vi "Build Measurement.vi"() -> ()   [LabVIEW 2021]
uses:
  <vilib>/Utility/miscctls.llb/LVRowAndColumnTypeDef.ctl
  _Measurement Packager Utility/Packager Helpers/Queue Driver/controls/Queue Operations.ctl
  _Measurement Packager Utility/Packager Helpers/controls/Config File Operations.ctl
  _Measurement Packager Utility/Packager Helpers/controls/Data Holder.ctl
  <vilib>/Utility/miscctls.llb/LVPoint32TypeDef.ctl
  _Measurement Packager Utility/Packager Helpers/controls/Build Spec Details.ctl
  <vilib>/AppBuilder/AB_API_Simple/Get Build Specification Version (path).vi
  _Measurement Packager Utility/Packager Helpers/Queue Driver/Queue Driver.lvlib
  _Measurement Packager Utility/Packager Helpers/Packager Helpers.lvlib
  _Measurement Packager Utility/Packager Helpers/Dictionary/Dictionary.lvlib
  <vilib>/AppBuilder/AB_API_Simple/NI_App_Builder_API.lvlib
panel:
  out "error out":errorcluster
  out "Tab Control":T1(tab)
  in  "Open Directory":bool
  in  "Feed Path":path
  out "Warning":bool=TRUE caption="Feed Path cannot be empty/invalid"
  in  "Next to select":bool
  in  "Build Package":bool
  in  "Project":path caption="LabVIEW Project Path"
  in  "Feed":T2(radio)
  in  "Back 1":bool
  in  "Populate Package":bool
  in  "Select All":bool
  out "Measurement List":i32(listbox)=-1 caption="Select the Measurements to build the package"
  out "Selection warning":string="Selected Project doesn't have EXE build spec"
  out "Maintainer Warning":string
  in  "Settings Page":enum32{"Page 1", "Page 2"}(tab)
  in  "Maintainer Email ID":string="sabthagiri@ni.com"
  in  "Architecture":string(combo)="1"
  in  "Maintainer":string="NI"
  in  "Back 2":bool
  in  "Start Build":bool
  in  "Package List":i32[](listbox) caption="Edit the Package Name and Version"
  in  "Settings":bool
  in  "Progres Bar":i32(slide)=9 caption="Creating Distribution..." scale=0.0..100.0
  in  "Start Next":bool
  in  "Log":bool[](array[boolean])=[TRUE, TRUE]
  in  "Build Status":i32(listbox)=-1
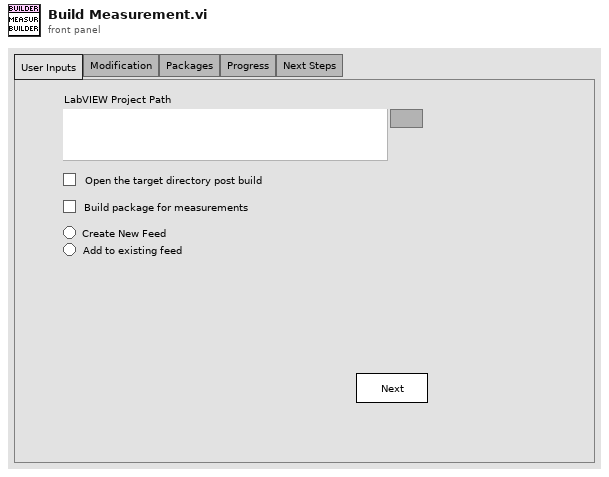
[diagram p1: front panel]
types:
  T1 = enum32{"User Inputs", "Modification", "Packages", "Progress", "Next Steps"}
  T2 = enum32{"No Selection", "CreateFeed", "AddtoFeed"}
  T3 = typedef "Queue Driver.lvlib/Queue Operations.ctl" = enum16{"Create Q", "Enqueue", "Enqueue N", "Dequeue", "Flush", "Release"}
  T4 = typedef "LVRowAndColumnTypeDef.ctl" = cluster{"Row":i32, "Column":i32}
  T5 = enum8{"Enabled", "Disabled", "Disabled and Grayed Out"}
  T6 = typedef "Packager Helpers.lvlib/Config File Operations.ctl" = enum16{"Read", "Write"}
  T7 = typedef "Packager Helpers.lvlib/Data Holder.ctl" = cluster{"Next Clicked?":bool, "MosueDown Coords":T8, "Build Spec":T9[], "No of Meas":i32, "No. of Selected Meas":i32, "Selected Meas":T9[], "Package Details":string[][], "Build Packge?":bool, "Packages Path":path, "Feed":enum32{"No Selection", "CreateFeed", "AddtoFeed"}, "Feed Path":path, "Valid Inputs?":bool, "Feed Old":enum32{"No Selection", "CreateFeed", "AddtoFeed"}, "Status":string[], "Open Directory?":bool}
  T8 = typedef "LVPoint32TypeDef.ctl" = cluster{"Horizontal":i32, "Vertical":i32}
  T9 = typedef "Packager Helpers.lvlib/Build Spec Details.ctl" = cluster{"EXE Name":string, "Target path":path, "Has PPL?":bool, "PPL Name":string}
  T10 = typedef "NI_App_Builder_API.lvlib/Build Specification Version.ctl" = cluster{"Major":u16, "Minor":u16, "Fix":u16, "Build":u16}
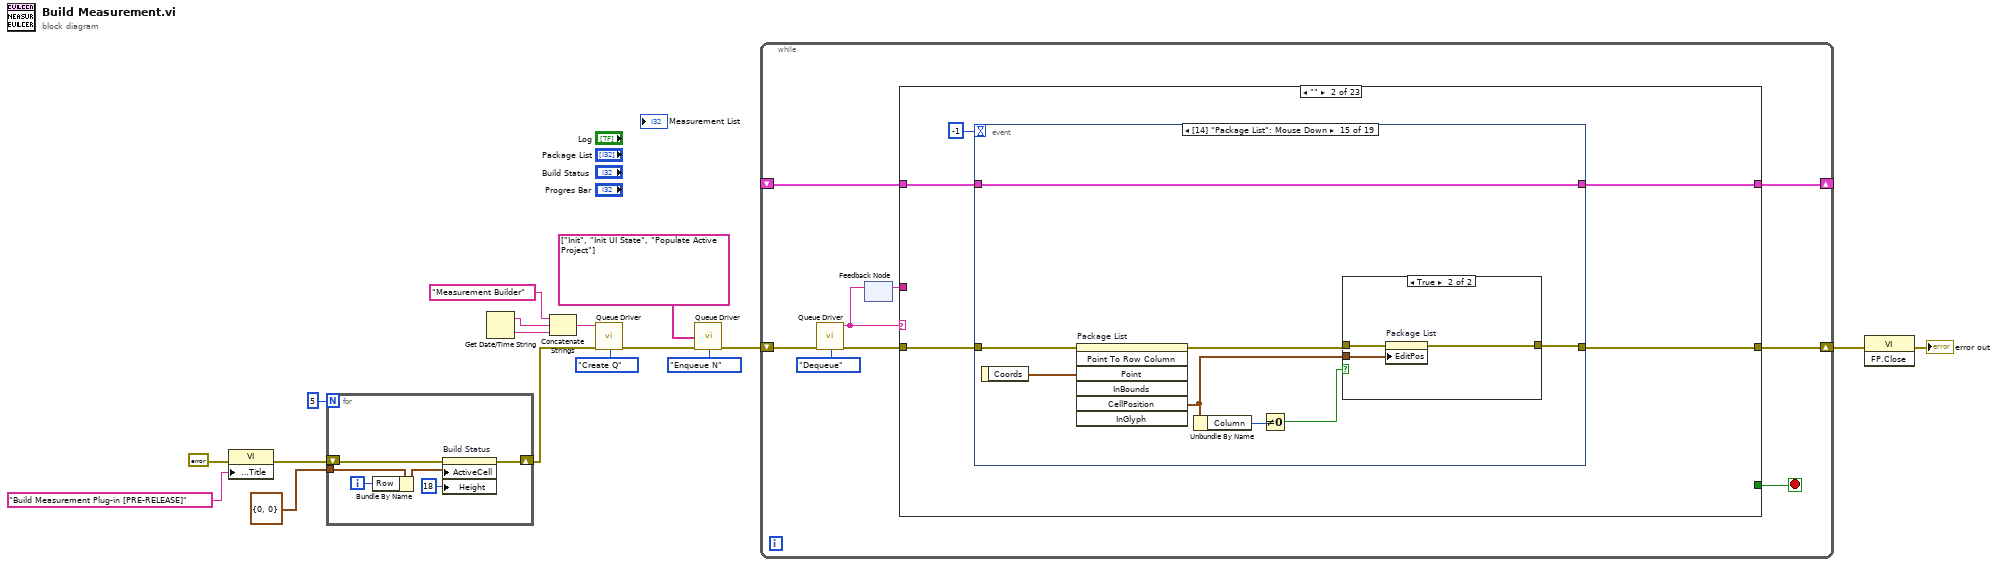
[diagram p0: block diagram]
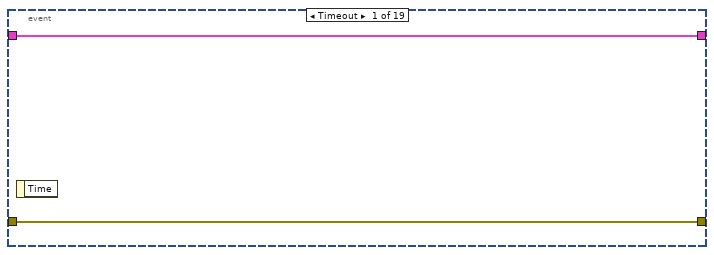
[diagram p3: hidden frame]
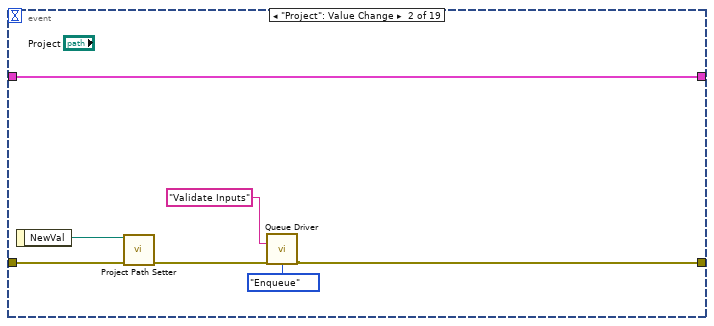
[diagram p4: hidden frame]
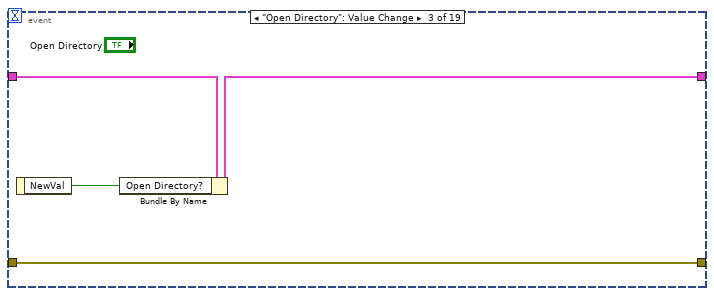
[diagram p5: hidden frame]
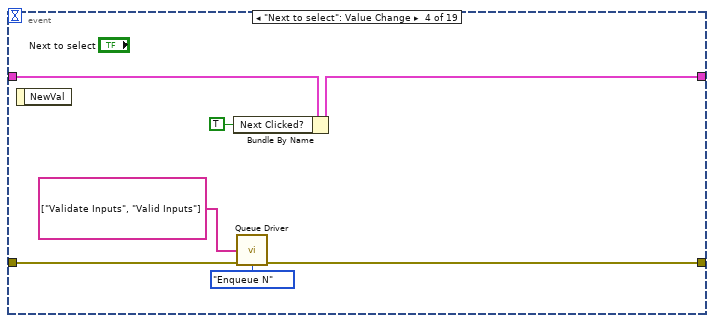
[diagram p6: hidden frame]
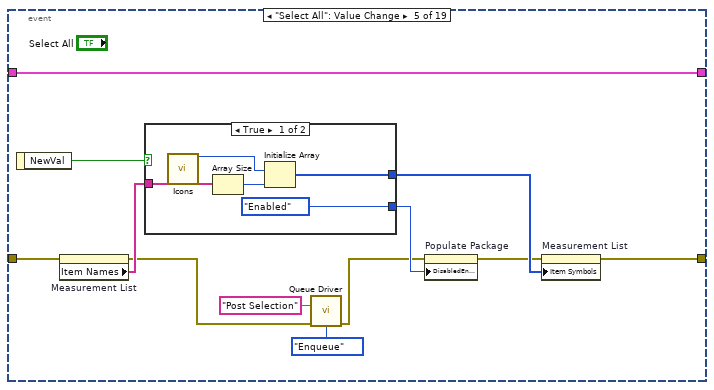
[diagram p7: hidden frame]
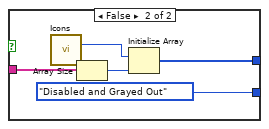
[diagram p8: hidden frame]
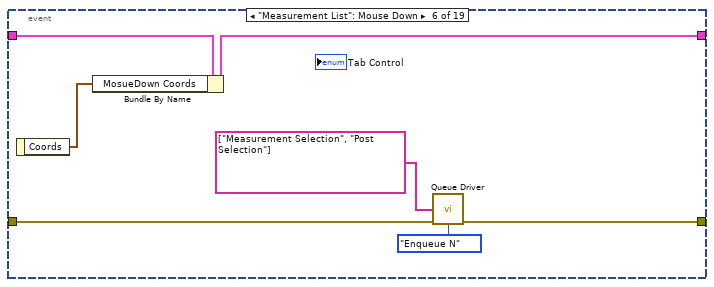
[diagram p9: hidden frame]
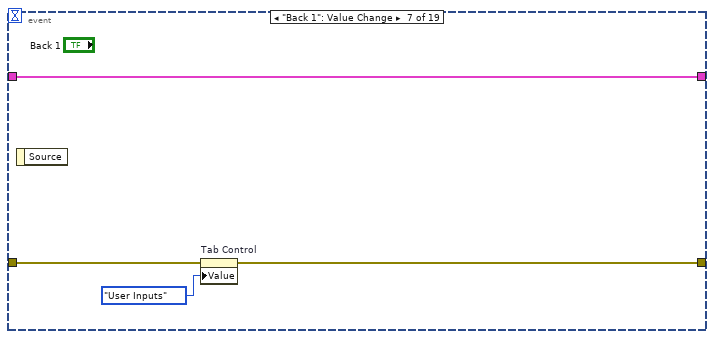
[diagram p10: hidden frame]
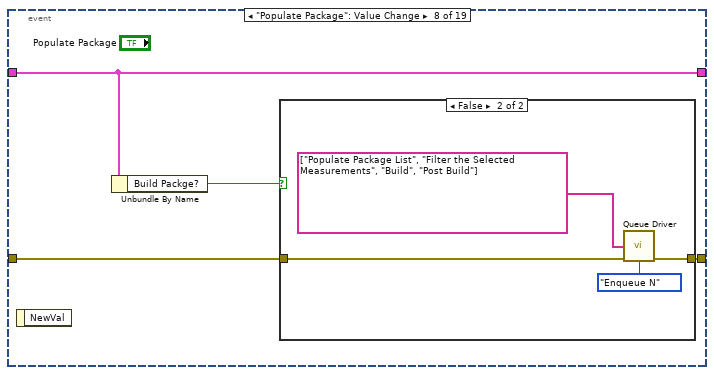
[diagram p11: hidden frame]
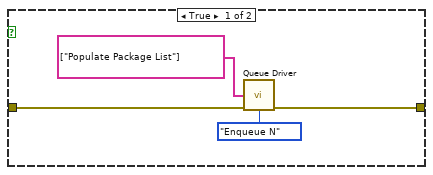
[diagram p12: hidden frame]
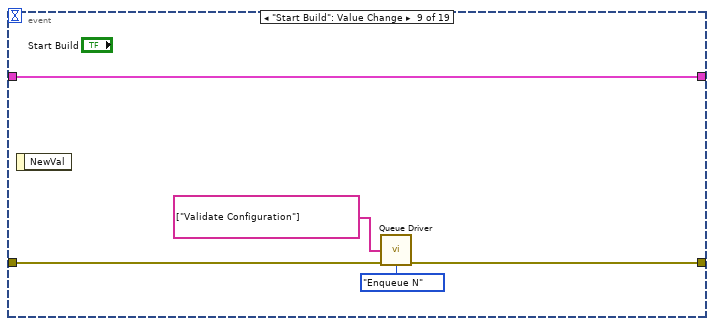
[diagram p13: hidden frame]
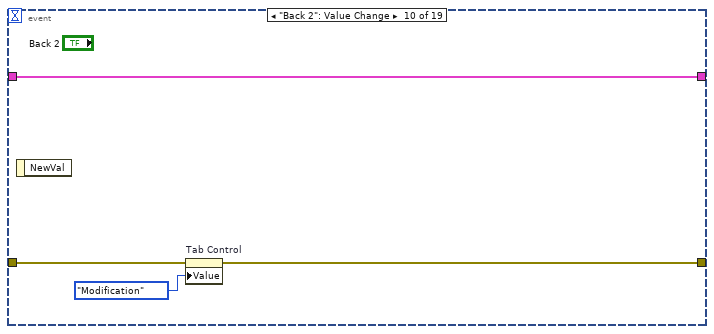
[diagram p14: hidden frame]
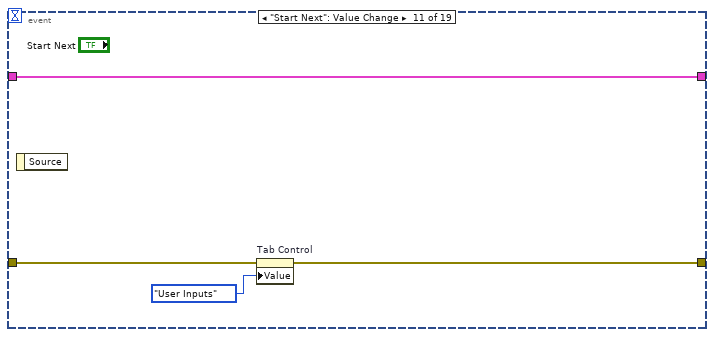
[diagram p15: hidden frame]
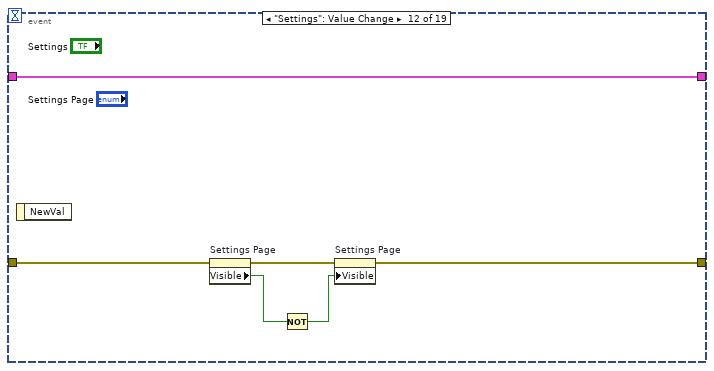
[diagram p16: hidden frame]
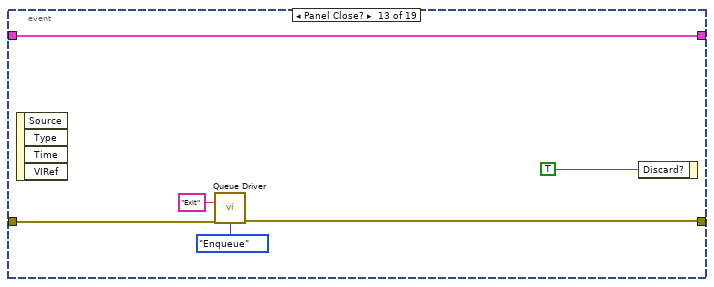
[diagram p17: hidden frame]
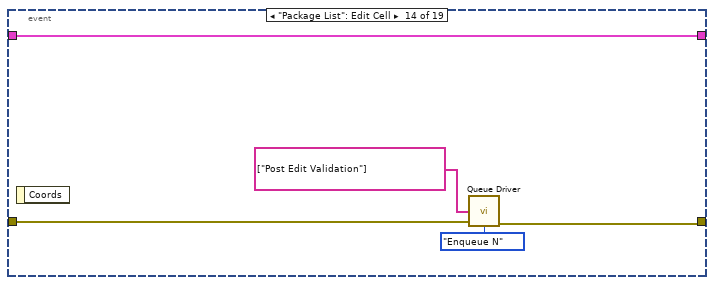
[diagram p18: hidden frame]
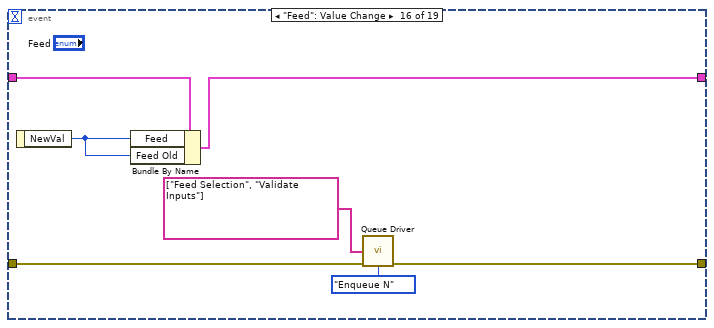
[diagram p20: hidden frame]
diagram:
  n1 = property class="VI"(error in=errorcluster {"status"=FALSE, "code"=0, "source"=""} ("error in (no error)"), "Front Panel.Title"="Build Measurement Plug-in [PRE-RELEASE]" ("Front Panel Window:Title")) -> (error out=w3:errorcluster)  [unwired: 1 in, 1 out]
  n2 = for {
    N: 5 -> [_]
    tunnel: T4 {"Row"=0, "Column"=0} ("Active Cell:Active Cell") -> [w23]
    shift-right: [w19] -> w6
    shift-left: w3 -> [w18]
    i -> [w21]
    n3 = Bundle By Name(cluster=w23, "Row"=w21) -> (w22:T4)
    n4 = property on="Build Status" class="MCListbox (strict)"(error in=w18, "ActiveCell"=w22, "Height"=u32 18 ("Active Cell:Cell Size:Height")) -> (error out=w19:errorcluster)  [unwired: 1 in, 1 out]
  }
  n5 = Get Date/Time String() -> (date string=w9:string, time string=w10:string)  [unwired: 3 in]
  n6 = Concatenate Strings("Measurement Builder" ("string"), w9, w10) -> (w7:string)
  n7 = call "Queue Driver.vi"("Name"=w7, "error in (no error)"=w6, "Q Operations"=Queue_Operations."Create Q") -> ("error out"=w13:errorcluster)  [unwired: 11 in, 1 out]
  n8 = call "Queue Driver.vi"("States[]"=string[] ["Init", "Init UI State", "Populate Active Project"], "error in (no error)"=w13, "Q Operations"=Queue_Operations."Enqueue N") -> ("error out"=w15:errorcluster)  [unwired: 11 in, 1 out]
  n9 = while {
    shift-right: [w29] -> w5
    shift-left: w15 -> [w32]
    shift-right: [w27] -> _
    shift-left: _ -> [w26]
    stop <- w28 stop-if-true
    n10 = call "Queue Driver.vi"("error in (no error)"=w32, "Q Operations"=Queue_Operations."Dequeue") -> ("Dequeued State"=w25:string, "error out"=w30:errorcluster)  [unwired: 12 in]
    n11 = feedback #1() -> (w24:string)  [unwired: 1 in]
    n12 = feedback-in #1(w25) -> ()
    n13 = case shown="\"\"" w25 {
      tunnel: w30 -> [w34 w38 w179 w194 w213 w225 w242 w291 w306 w328 w342 w367 w393 w399 w408 w433 w462 w472 w487 w506 w509 w526 w532]
      tunnel: [w34 w39 w176 w188 w206 w224 w239 w290 w309 w326 w338 w359 w388 w400 w405 w427 w461 w468 w478 w507 w515 w525 w531] -> w29
      tunnel: [_ _ _ _ _ _ _ _ _ _ _ _ _ _ _ _ _ _ _ _ _ _ TRUE] -> w28
      tunnel: [w33 w36 w178 w190 w209 w226 w238 w289 w311 w329 w345 w368 w391 w401 w412 w424 w463 w464 w488 w505 w514 w527 w528] -> w27
      tunnel: w26 -> [w33 w35 _ w190 w210 w226 w237 w289 w312 w329 w345 w368 w394 w401 w412 w421 w463 w466 w488 w499 w514 w527 w528]
      tunnel: w24 -> [_ _ _ _ _ _ _ _ _ _ _ _ _ _ _ _ _ _ _ _ _ _ _]
      frame Default {
      }
      frame "" {
        n14 = event shown="[14] \"Package List\": Mouse Down" {
          selector: _ -> [_ _ _ _ _ _ _ _ _ _ _ _ _ _ _ _ _ _ _]
          dyn-events: _ -> [_ _ _ _ _ _ _ _ _ _ _ _ _ _ _ _ _ _ _]
          timeout: -1 -> [_ _ _ _ _ _ _ _ _ _ _ _ _ _ _ _ _ _ _]
          tunnel: [w41 w44 w52 w58 w64 w85 w91 w95 w107 w112 w116 w120 w127 w132 w135 w150 w156 w165 w168] -> w39
          tunnel: w38 -> [w41 w48 w52 w59 w69 w87 w92 w96 w108 w113 w117 w121 w128 w130 w140 w149 w155 w164 w169]
          tunnel: [w40 w42 w50 w55 w71 w84 w90 w94 w109 w111 w115 w118 w124 w134 w142 w152 w159 w167 w173] -> w36
          tunnel: w35 -> [w40 w42 w51 w56 w71 w88 w90 w94 w109 w111 w115 w118 w124 w134 w142 w153 w160 w167 w174]
          event Timeout {
            n15 = event-data() -> ()  [unwired: 1 in, 1 out]
          }
          event "Project": Value Change {
            n16 = event-data() -> ("NewVal"=w47:path)  [unwired: 1 in]
            n17 = call "Project Path Setter.vi"("ProjectPath In"=w47, "error in (no error)"=w48) -> ("error out"=w43:errorcluster)  [unwired: 13 in]
            n18 = call "Queue Driver.vi"("State"="Validate Inputs", "error in (no error)"=w43, "Q Operations"=Queue_Operations."Enqueue") -> ("error out"=w44:errorcluster)  [unwired: 11 in, 1 out]
          }
          event "Open Directory": Value Change {
            n19 = event-data() -> ("NewVal"=w49:bool)  [unwired: 1 in]
            n20 = Bundle By Name(cluster=w51, "Open Directory?"=w49) -> (w50:T7)
          }
          event "Next to select": Value Change {
            n21 = event-data() -> ()  [unwired: 1 in, 1 out]
            n22 = Bundle By Name(cluster=w56, "Next Clicked?"=TRUE) -> (w55:T7)
            n23 = call "Queue Driver.vi"("States[]"=string[] ["Validate Inputs", "Valid Inputs"], "error in (no error)"=w59, "Q Operations"=Queue_Operations."Enqueue N") -> ("error out"=w58:errorcluster)  [unwired: 11 in, 1 out]
          }
          event "Select All": Value Change {
            n24 = event-data() -> ("NewVal"=w70:bool)  [unwired: 1 in]
            n25 = property on="Measurement List" class="LstBox (strict)"(error in=w69) -> (error out=w61:errorcluster, "Item Names"=w68:string[])  [unwired: 1 in, 1 out]
            n26 = case shown="True" w70 {
              tunnel: w68 -> [w75 w80]
              tunnel: [w74 w79] -> w67
              tunnel: [T5."Enabled" ("Disabled") T5."Disabled and Grayed Out" ("Disabled")] -> w66
              frame True {
                n27 = call "Icons.vi"() -> ("Selected"=w72:i32)  [unwired: 14 in, 1 out]
                n28 = Array Size(array=w75) -> (size(s)=w76:i32)
                n29 = Initialize Array(w72, w76) -> (w74:i32[])
              }
              frame False {
                n30 = call "Icons.vi"() -> ("Non Selected"=w77:i32)  [unwired: 14 in, 1 out]
                n31 = Array Size(array=w80) -> (size(s)=w81:i32)
                n32 = Initialize Array(w77, w81) -> (w79:i32[])
              }
            }
            n33 = call "Queue Driver.vi"("State"="Post Selection", "error in (no error)"=w61, "Q Operations"=Queue_Operations."Enqueue") -> ("error out"=w60:errorcluster)  [unwired: 11 in, 1 out]
            n34 = property on="Populate Package" class="Bool"(error in=w60, "DisabledEnum"=w66) -> (error out=w65:errorcluster)  [unwired: 1 in, 1 out]
            n35 = property on="Measurement List" class="LstBox (strict)"(error in=w65, "Item Symbols"=w67) -> (error out=w64:errorcluster)  [unwired: 1 in, 1 out]
          }
          event "Measurement List": Mouse Down {
            n36 = event-data() -> ("Coords"=w82:T8)  [unwired: 1 in]
            n37 = Bundle By Name(cluster=w88, "MosueDown Coords"=w82) -> (w84:T7)
            n38 = call "Queue Driver.vi"("States[]"=string[] ["Measurement Selection", "Post Selection"], "error in (no error)"=w87, "Q Operations"=Queue_Operations."Enqueue N") -> ("error out"=w85:errorcluster)  [unwired: 11 in, 1 out]
          }
          event "Back 1": Value Change {
            n39 = event-data() -> ()  [unwired: 1 in, 1 out]
            n40 = property on="Tab Control" class="TabCtl (strict)"(error in=w92, "Value"=T1."User Inputs" ("Tab Control")) -> (error out=w91:errorcluster)  [unwired: 1 in, 1 out]
          }
          event "Populate Package": Value Change {
            n41 = event-data() -> ()  [unwired: 1 in, 1 out]
            n42 = Unbundle By Name(w94) -> ("Build Packge?"=w93:bool)
            n43 = case shown="False" w93 {
              tunnel: w96 -> [w100 w104]
              tunnel: [w99 w103] -> w95
              frame True {
                n44 = call "Queue Driver.vi"("States[]"=string[] ["Populate Package List"], "error in (no error)"=w100, "Q Operations"=Queue_Operations."Enqueue N") -> ("error out"=w99:errorcluster)  [unwired: 11 in, 1 out]
              }
              frame False {
                n45 = call "Queue Driver.vi"("States[]"=string[] ["Populate Package List", "Filter the Selected Measurements", "Build", "Post Build"], "error in (no error)"=w104, "Q Operations"=Queue_Operations."Enqueue N") -> ("error out"=w103:errorcluster)  [unwired: 11 in, 1 out]
              }
            }
          }
          event "Start Build": Value Change {
            n46 = event-data() -> ()  [unwired: 1 in, 1 out]
            n47 = call "Queue Driver.vi"("States[]"=string[] ["Validate Configuration"], "error in (no error)"=w108, "Q Operations"=Queue_Operations."Enqueue N") -> ("error out"=w107:errorcluster)  [unwired: 11 in, 1 out]
          }
          event "Back 2": Value Change {
            n48 = event-data() -> ()  [unwired: 1 in, 1 out]
            n49 = property on="Tab Control" class="TabCtl (strict)"(error in=w113, "Value"=T1."Modification" ("Tab Control")) -> (error out=w112:errorcluster)  [unwired: 1 in, 1 out]
          }
          event "Start Next": Value Change {
            n50 = event-data() -> ()  [unwired: 1 in, 1 out]
            n51 = property on="Tab Control" class="TabCtl (strict)"(error in=w117, "Value"=T1."User Inputs" ("Tab Control")) -> (error out=w116:errorcluster)  [unwired: 1 in, 1 out]
          }
          event "Settings": Value Change {
            n52 = event-data() -> ()  [unwired: 1 in, 1 out]
            n53 = property on="Settings Page" class="TabCtl (strict)"(error in=w121) -> (error out=w119:errorcluster, "Visible"=w123:bool)  [unwired: 1 in, 1 out]
            n54 = Not(x=w123) -> (.not. x?=w122:bool)
            n55 = property on="Settings Page" class="TabCtl (strict)"(error in=w119, "Visible"=w122) -> (error out=w120:errorcluster)  [unwired: 1 in, 1 out]
          }
          event Panel Close? {
            n56 = event-data() -> ()  [unwired: 1 in, 4 out]
            n57 = call "Queue Driver.vi"("State"="Exit", "error in (no error)"=w128, "Q Operations"=Queue_Operations."Enqueue") -> ("error out"=w127:errorcluster)  [unwired: 11 in, 1 out]
            n58 = event-data("Discard?"=TRUE) -> ()  [unwired: 1 in, 1 out]
          }
          event "Package List": Edit Cell {
            n59 = event-data() -> ()  [unwired: 1 in, 1 out]
            n60 = call "Queue Driver.vi"("States[]"=string[] ["Post Edit Validation"], "error in (no error)"=w130, "Q Operations"=Queue_Operations."Enqueue N") -> ("error out"=w132:errorcluster)  [unwired: 11 in, 1 out]
          }
          event "Package List": Mouse Down {
            n61 = event-data() -> ("Coords"=w141:T8)  [unwired: 1 in]
            n62 = invoke on="Package List" class="MCListbox (strict)" method="Point To Row Column"(error in=w140, "Point"=w141) -> (error out=w139:errorcluster, "CellPosition"=w136:T4)  [unwired: 5 in, 5 out]
            n63 = Unbundle By Name(w136) -> ("Column"=w138:i32)
            n64 = Not Equal To 0?(x=w138) -> (x != 0?=w137:bool)
            n65 = case shown="True" w137 {
              tunnel: w139 -> [w143 w146]
              tunnel: [w143 w145] -> w135
              tunnel: w136 -> [_ w144]
              frame False {
              }
              frame True {
                n66 = property on="Package List" class="MCListbox (strict)"(error in=w146, "EditPos"=w144) -> (error out=w145:errorcluster)  [unwired: 1 in, 1 out]
              }
            }
          }
          event "Feed": Value Change {
            n67 = event-data() -> ("NewVal"=w147:T2)  [unwired: 1 in]
            n68 = Bundle By Name(cluster=w153, "Feed"=w147, "Feed Old"=w147) -> (w152:T7)
            n69 = call "Queue Driver.vi"("States[]"=string[] ["Feed Selection", "Validate Inputs"], "error in (no error)"=w149, "Q Operations"=Queue_Operations."Enqueue N") -> ("error out"=w150:errorcluster)  [unwired: 11 in, 1 out]
          }
          event "Build Package": Value Change {
            n70 = event-data() -> ("NewVal"=w158:bool)  [unwired: 1 in]
            n71 = Bundle By Name(cluster=w160, "Build Packge?"=w158) -> (w159:T7)
            n72 = call "Queue Driver.vi"("States[]"=string[] ["Build Package Value Change", "Validate Inputs"], "error in (no error)"=w155, "Q Operations"=Queue_Operations."Enqueue N") -> ("error out"=w156:errorcluster)  [unwired: 11 in, 1 out]
          }
          event "Architecture", "Maintainer", "Maintainer Email ID": Value Change {
            n73 = event-data() -> ()  [unwired: 1 in, 1 out]
            n74 = call "Read or Write Configurations.vi"("Architecture"="Architecture", "Maintainer"="Maintainer", "Email"="Maintainer Email ID", "error in (no error)"=w164, "Operation"=Config_File_Operations."Write") -> ("error out"=w165:errorcluster)  [unwired: 7 in, 3 out]
          }
          event "Feed Path": Value Change {
            n75 = event-data() -> ("NewVal"=w172:path)  [unwired: 1 in]
            n76 = Bundle By Name(cluster=w174, "Feed Path"=w172) -> (w173:T7)
            n77 = call "Queue Driver.vi"("States[]"=string[] ["Validate Inputs"], "error in (no error)"=w169, "Q Operations"=Queue_Operations."Enqueue N") -> ("error out"=w168:errorcluster)  [unwired: 11 in, 1 out]
          }
        }
      }
      frame "Init" {
        w177 = TRUE ("Open Directory?")
        n78 = invoke class="VI" method="Default Vals.Reinit All"(error in=w179) -> (error out=w175:errorcluster)  [unwired: 2 in, 2 out]
        n79 = property on="Open Directory" class="Bool (strict)"(error in=w175, "Value"=w177) -> (error out=w176:errorcluster)  [unwired: 1 in, 1 out]
        n80 = Bundle By Name(cluster=T7 {"Next Clicked?"=TRUE, "MosueDown Coords"={"Horizontal"=0, "Vertical"=0}, "Build Spec"=[], "No of Meas"=0, "No. of Selected Meas"=0, "Selected Meas"=[], "Package Details"=[], "Build Packge?"=FALSE, "Packages Path"=path "", "Feed"=enum."No Selection", "Feed Path"=path "", "Valid Inputs?"=FALSE, "Feed Old"=enum."No Selection", "Status"=[], "Open Directory?"=FALSE}, "Open Directory?"=w177) -> (w178:T7)
      }
      frame "Init UI State" {
        w187 = u32 16448250 ("Selection Color")
        w184 = FALSE ("Visible")
        n81 = property on="Tab Control" class="TabCtl (strict)"(error in=w194, "Value"=T1."User Inputs" ("Tab Control")) -> (error out=w197:errorcluster)  [unwired: 1 in, 1 out]
        n82 = property on="Settings Page" class="TabCtl (strict)"(error in=w197, "Visible"=w184) -> (error out=w196:errorcluster)  [unwired: 1 in, 1 out]
        n83 = property on="Warning" class="Bool"(error in=w196, "Visible"=w184) -> (error out=w181:errorcluster)  [unwired: 1 in, 1 out]
        n84 = property on="Selection warning" class="Str"(error in=w181, "Visible"=w184) -> (error out=w186:errorcluster)  [unwired: 1 in, 1 out]
        n85 = property on="Feed Path" class="Path"(error in=w186, "Visible"=w184) -> (error out=w185:errorcluster)  [unwired: 1 in, 1 out]
        n86 = property on="Settings" class="Bool"(error in=w185, "Visible"=w184) -> (error out=w183:errorcluster)  [unwired: 1 in, 1 out]
        n87 = property on="Measurement List" class="LstBox (strict)"(error in=w183, "SelColor"=w187) -> (error out=w195:errorcluster)  [unwired: 1 in, 1 out]
        n88 = property on="Package List" class="MCListbox (strict)"(error in=w195, "SelColor"=w187) -> (error out=w189:errorcluster)  [unwired: 1 in, 1 out]
        n89 = property on="Build Status" class="MCListbox (strict)"(error in=w189, "SelColor"=w187) -> (error out=w188:errorcluster)  [unwired: 1 in, 1 out]
        "Selection warning" <- "Atleast one measurement should be selected" ("Selection warning")
        "Maintainer Warning" <- "Maintainer and Email ID cannot be empty" ("Maintainer Warning")
        "Warning" <- TRUE ("Warning")
      }
      frame "Populate Active Project" {
        # "Get the active labview project"
        n90 = call "Get Active ProjectPath.vi"("error in (no error)"=w213) -> ("Project Path"=w201:path, "error out"=w212:errorcluster)  [unwired: 13 in]
        n91 = property on="Project" class="Path"(error in=w212, "Value"=w201) -> (error out=w211:errorcluster)  [unwired: 1 in, 1 out]
        n92 = call "Project Path Setter.vi"("ProjectPath In"=w201, "error in (no error)"=w211) -> ("error out"=w208:errorcluster)  [unwired: 13 in]
        n93 = Empty String/Path?(string/path=w201) -> (empty?=w200:bool)
        n94 = Not A Number/Path/Refnum?(number/path/refnum=w201) -> (NaN/Path/Refnum?=w199:bool)
        n95 = Or(x=w199, y=w200) -> (x .or. y?=w198:bool)
        n96 = case "Not a valid path?" shown="False" w198 {
          tunnel: w210 -> [w218 w223]
          tunnel: [w217 w222] -> w209
          tunnel: [w215 w221] -> w207
          tunnel: [T5."Disabled and Grayed Out" ("Disabled") T5."Enabled" ("Disabled")] -> w204
          frame True {
            w215 = T2."No Selection" ("Feed")
            n97 = Bundle By Name(cluster=w218, "Build Packge?"=FALSE, "Feed"=w215) -> (w217:T7)
          }
          frame False {
            w221 = T2."CreateFeed" ("Feed")
            n98 = Bundle By Name(cluster=w223, "Build Packge?"=TRUE, "Feed"=w221) -> (w222:T7)
          }
        }
        n99 = Not(x=w198) -> (.not. x?=w205:bool)
        n100 = property on="Build Package" class="Bool (strict)"(error in=w208, "Value"=w205) -> (error out=w203:errorcluster)  [unwired: 1 in, 1 out]
        n101 = property on="Feed" class="RadioBtnsControl (strict)"(error in=w203, "DisabledEnum"=w204) -> (error out=w202:errorcluster)  [unwired: 1 in, 1 out]
        n102 = property on="Feed" class="RadioBtnsControl (strict)"(error in=w202, "Value"=w207) -> (error out=w206:errorcluster)  [unwired: 1 in, 1 out]
      }
      frame "Populate Config" {
        # "Disabling it because the config will not be populated in UI"
        # "Populate Config Data"
        n103 = disable-structure shown="Disabled" {
          disable-tunnel: w225 -> [w235 w236]
          disable-tunnel: [w227 w236] -> w224
          frame Disabled {
            n104 = call "Read or Write Configurations.vi"("error in (no error)"=w235, "Operation"=Config_File_Operations."Read") -> ("Architecture OUT"=w233:string, "Maintainer OUT"=w232:string, "Email OUT"=w231:string, "error out"=w230:errorcluster)  [unwired: 10 in]
            n105 = property on="Maintainer Email ID" class="Str"(error in=w230, "Value"=w231) -> (error out=w229:errorcluster)  [unwired: 1 in, 1 out]
            n106 = property on="Maintainer" class="Str"(error in=w229, "Value"=w232) -> (error out=w228:errorcluster)  [unwired: 1 in, 1 out]
            n107 = property on="Architecture" class="CmbBox"(error in=w228, "Value"=w233) -> (error out=w227:errorcluster)  [unwired: 1 in, 1 out]
          }
          frame Enabled {
          }
        }
      }
      frame "Validate Inputs" {
        # "Validate Inputs"
        n108 = call "Validate Project Path.vi"("error in (no error)"=w242) -> ("Valid Path?"=w241:bool, "error out"=w240:errorcluster)  [unwired: 13 in]
        n109 = case "Valid project?" shown="False" w241 {
          tunnel: w240 -> [w248 w256]
          tunnel: [w247 w251] -> w239
          tunnel: [w244 w252] -> w238
          tunnel: w237 -> [w245 w253]
          frame False {
            n110 = property on="Warning" class="Bool"(error in=w248, "Visible"=TRUE, "Caption.Text"="Existing LabVIEW Project Path should be selected" ("Boolean Text.Text")) -> (error out=w247:errorcluster)  [unwired: 1 in, 1 out]
            n111 = Bundle By Name(cluster=w245, "Valid Inputs?"=FALSE) -> (w244:T7)
          }
          frame True {
            n112 = Unbundle By Name(w253) -> ("Build Packge?"=w250:bool, "Feed"=w255:T2, "Feed Path"=w254:path)
            n113 = case "Build package ?" shown="True" w250 {
              tunnel: w256 -> [w258 w268]
              tunnel: w255 -> [_ w267]
              tunnel: w254 -> [_ w266]
              tunnel: w253 -> [w261 w265]
              tunnel: [w260 w264] -> w252
              tunnel: [w262 w263] -> w251
              frame False {
                # "Invalid project Path"
                n114 = Bundle By Name(cluster=w261, "Valid Inputs?"=TRUE) -> (w260:T7)
                n115 = property on="Warning" class="Bool"(error in=w258, "Visible"=FALSE) -> (error out=w262:errorcluster)  [unwired: 1 in, 1 out]
              }
              frame True {
                n116 = case shown="Default" w267 {
                  tunnel: w268 -> [w275 w283]
                  tunnel: w266 -> [w276 _]
                  tunnel: w265 -> [w281 w287]
                  tunnel: [w280 w286] -> w264
                  tunnel: [w278 w282] -> w263
                  frame "AddtoFeed" {
                    # "Validate Path"
                    n117 = Empty String/Path?(string/path=w276) -> (empty?=w274:bool)
                    n118 = call <vilib>:"Check if File or Folder Exists.vi"("error in (no error)"=w275, "path"=w276) -> ("error out"=w270:errorcluster, "file or folder exists?"=w272:bool)  [unwired: 7 in, 1 out]
                    n119 = Not A Number/Path/Refnum?(number/path/refnum=w276) -> (NaN/Path/Refnum?=w273:bool)
                    n120 = Or(x=w274, y=w273) -> ()  [unwired: 1 out]
                    n121 = Not(x=w272) -> (.not. x?=w269:bool)
                    n122 = Compound Arithmetic op=OR(w274, w273, w269) -> (w271:bool)
                    n123 = Not(x=w271) -> (.not. x?=w277:bool)
                    n124 = Bundle By Name(cluster=w281, "Valid Inputs?"=w277) -> (w280:T7)
                    n125 = property on="Warning" class="Bool"(error in=w270, "Visible"=w271, "Caption.Text"="Feed Path cannot be empty/invalid" ("Boolean Text.Text")) -> (error out=w278:errorcluster)  [unwired: 1 in, 1 out]
                  }
                  frame Default {
                    n126 = property on="Warning" class="Bool"(error in=w283, "Visible"=FALSE) -> (error out=w282:errorcluster)  [unwired: 1 in, 1 out]
                    n127 = Bundle By Name(cluster=w287, "Valid Inputs?"=TRUE) -> (w286:T7)
                  }
                }
              }
            }
          }
        }
      }
      frame "Valid Inputs" {
        # "Check if valid inputs and if next is clicked"
        n128 = Unbundle By Name(w289) -> ("Valid Inputs?"=w288:bool)
        n129 = case "Valid Inputs?" shown="True" w288 {
          tunnel: w291 -> [w292 w298]
          tunnel: [w292 w294] -> w290
          tunnel: w289 -> [_ w293]
          frame False {
          }
          frame True {
            n130 = Unbundle By Name(w293) -> ("Next Clicked?"=w295:bool)
            n131 = property on="Warning" class="Bool"(error in=w298, "Visible"=FALSE) -> (error out=w296:errorcluster)  [unwired: 1 in, 1 out]
            n132 = case "Next Clicked?" shown="True" w295 {
              tunnel: w296 -> [w299 w302]
              tunnel: [w299 w300] -> w294
              frame False {
              }
              frame True {
                n133 = call "Queue Driver.vi"("States[]"=string[] ["Populate Measurements", "Update Tab", "Validate Measurement"], "error in (no error)"=w302, "Q Operations"=Queue_Operations."Enqueue N") -> ("error out"=w300:errorcluster)  [unwired: 11 in, 1 out]
              }
            }
          }
        }
      }
      frame "Build Package Value Change" {
        # "Build Package Value Change Handling"
        n134 = Unbundle By Name(w312) -> ("Feed"=w305:T2, "Build Packge?"=w313:bool, "Feed Old"=w308:T2)
        n135 = case shown="False" w313 {
          tunnel: w312 -> [w318 w324]
          tunnel: [w317 w321] -> w311
          tunnel: [T5."Disabled and Grayed Out" ("Disabled") T5."Enabled" ("Disabled")] -> w314
          tunnel: w308 -> [w315 w320]
          tunnel: [_ w322] -> w307
          tunnel: w305 -> [w316 _]
          tunnel: [w315 w320] -> w304
          frame False {
            n136 = Bundle By Name(cluster=w318, "Feed Old"=w316) -> (w317:T7)
          }
          frame True {
            n137 = case shown="\"AddtoFeed\"" w320 {
              tunnel: [TRUE _] -> w322
              frame "AddtoFeed" {
              }
              frame Default {
              }
            }
            n138 = Bundle By Name(cluster=w324, "Feed"=w320) -> (w321:T7)
          }
        }
        n139 = property on="Feed Path" class="Path"(error in=w306, "Visible"=w307) -> (error out=w310:errorcluster)  [unwired: 1 in, 1 out]
        n140 = property on="Feed" class="RadioBtnsControl (strict)"(error in=w310, "DisabledEnum"=w314, "Value"=w304) -> (error out=w309:errorcluster)  [unwired: 1 in, 1 out]
      }
      frame "Feed Selection" {
        # "Feed Selection Value Change Handling"
        n141 = Unbundle By Name(w329) -> ("Feed"=w327:T2)
        n142 = case shown="Default" w327 {
          tunnel: w328 -> [w331 w335]
          tunnel: [w330 w333] -> w326
          frame Default {
            n143 = property on="Feed Path" class="Path"(error in=w331, "Visible"=FALSE) -> (error out=w330:errorcluster)  [unwired: 1 in, 1 out]
          }
          frame "AddtoFeed" {
            n144 = property on="Feed Path" class="Path"(error in=w335, "Visible"=TRUE) -> (error out=w333:errorcluster)  [unwired: 1 in, 1 out]
          }
        }
      }
      frame "Measurement Selection" {
        # "Measurement Selection Value change"
        n145 = Unbundle By Name(w345) -> ("No of Meas"=w336:i32, "MosueDown Coords"=w344:T8)
        n146 = property on="Measurement List" class="LstBox (strict)"(error in=w342) -> (error out=w341:errorcluster, "Item Symbols"=w339:i32[])  [unwired: 1 in, 1 out]
        n147 = invoke on="Measurement List" class="LstBox (strict)" method="Point To Row"(error in=w341, "Point"=w344) -> (error out=w343:errorcluster, "Row"=w337:i32)  [unwired: 5 in, 5 out]
        n148 = Greater?(x=w336, y=w337) -> (0:w340:bool)
        n149 = case "Mouse click In range?" shown="True" w340 {
          tunnel: w343 -> [w346 w349]
          tunnel: w339 -> [_ w351]
          tunnel: [w346 w348] -> w338
          tunnel: w337 -> [_ w347]
          frame False {
          }
          frame True {
            # "Change the item symbols"
            n150 = in-place {
              n151 = in-place-array #2(w351, w347) -> (w355:i32)
              n152 = call "Icons.vi"() -> ("Selected"=w354:i32, "Non Selected"=w356:i32)  [unwired: 14 in]
              n153 = Equal?(x=w355, y=w354) -> (x = y?=w353:bool)
              n154 = Swap Values(12:w354, 13:w353, 14:w356) -> (1:w352:i32)  [unwired: 1 out]
              n155 = in-place-array #2(w352) -> (w350:i32[])  [unwired: 1 out]
            }
            n156 = property on="Measurement List" class="LstBox (strict)"(error in=w349, "Item Symbols"=w350) -> (error out=w348:errorcluster)  [unwired: 1 in, 1 out]
          }
        }
      }
      frame "Post Selection" {
        # "Selection change handling"
        n157 = property on="Measurement List" class="LstBox (strict)"(error in=w367) -> (error out=w364:errorcluster, "Item Symbols"=w366:i32[])  [unwired: 1 in, 1 out]
        n158 = call "Check the Symbols.vi"("Item Symbols"=w366) -> ("All Selected?"=w365:bool, "None Selected"=w363:bool)  [unwired: 13 in]
        n159 = case "All selected?" shown="False" w365 {
          tunnel: w364 -> [w372 w384]
          tunnel: w363 -> [w375 _]
          tunnel: [w373 T5."Enabled" ("Disabled")] -> w362
          tunnel: [w371 w381] -> w361
          tunnel: [w369 _] -> w358
          frame False {
            n160 = property on="Select All" class="Bool (strict)"(error in=w372, "Value"=FALSE ("All")) -> (error out=w370:errorcluster)  [unwired: 1 in, 1 out]
            n161 = case "None Selected?" shown="False" w375 {
              tunnel: [T5."Enabled" ("Disabled") T5."Disabled and Grayed Out" ("Disabled")] -> w373
              tunnel: [w376 w379] -> w371
              tunnel: w370 -> [w376 w379]
              tunnel: [_ TRUE] -> w369
              frame False {
              }
              frame True {
              }
            }
          }
          frame True {
            n162 = property on="Select All" class="Bool (strict)"(error in=w384, "Value"=TRUE ("All")) -> (error out=w381:errorcluster)  [unwired: 1 in, 1 out]
          }
        }
        n163 = property on="Populate Package" class="Bool"(error in=w361, "DisabledEnum"=w362) -> (error out=w360:errorcluster)  [unwired: 1 in, 1 out]
        n164 = property on="Selection warning" class="Str"(error in=w360, "Visible"=w358, "Value"="Atleast one measurement should be selected" ("Selection warning")) -> (error out=w359:errorcluster)  [unwired: 1 in, 1 out]
      }
      frame "Populate Measurements" {
        # "Populate the selected measurements with the package name"
        n165 = call "Get Measurement Names.vi"("error in (no error)"=w393) -> ("Build Details"=w390:T9[], "error out"=w392:errorcluster)  [unwired: 13 in]
        n166 = for {
          tunnel: w390 -> [w397] mode=indexing
          tunnel: [w396] -> w386 mode=indexing
          tunnel: [w395] -> w389 mode=indexing
          n167 = Unbundle By Name(w397) -> ("EXE Name"=w396:string)
          n168 = call "Icons.vi"() -> ("Selected"=w395:i32)  [unwired: 14 in, 1 out]
        }
        n169 = property on="Measurement List" class="LstBox (strict)"(error in=w392, "Item Names"=w386, "Item Symbols"=w389, "Active Row"=-1 ("Selection Mode")) -> (error out=w388:errorcluster)  [unwired: 1 in, 1 out]
        n170 = Array Size(array=w386) -> (size(s)=w385:i32)
        n171 = Bundle By Name(cluster=w394, "Build Spec"=w390, "No of Meas"=w385, "No. of Selected Meas"=w385) -> (w391:T7)
      }
      frame "Update Tab" {
        n172 = property on="Tab Control" class="TabCtl (strict)"(error in=w399, "Value"=T1."Modification" ("Tab Control")) -> (error out=w400:errorcluster)  [unwired: 1 in, 1 out]
      }
      frame "Validate Measurement" {
        # "Validate measurements"
        n173 = Unbundle By Name(w412) -> ("Build Spec"=w411:T9[])
        n174 = Empty Array?(array=w411) -> (empty?=w410:bool)
        n175 = case shown="False" w410 {
          tunnel: [T5."Enabled" ("Disabled") T5."Disabled and Grayed Out" ("Disabled")] -> w409
          tunnel: [TRUE ("All") FALSE ("All")] -> w404
          frame False {
          }
          frame True {
          }
        }
        n176 = property on="Populate Package" class="Bool"(error in=w408, "DisabledEnum"=w409) -> (error out=w407:errorcluster)  [unwired: 1 in, 1 out]
        n177 = property on="Select All" class="Bool (strict)"(error in=w407, "Value"=w404, "DisabledEnum"=w409) -> (error out=w406:errorcluster)  [unwired: 1 in, 1 out]
        n178 = Not(x=w404) -> (.not. x?=w403:bool)
        n179 = property on="Selection warning" class="Str"(error in=w406, "Visible"=w403, "Value"="Selected Project doesn't have EXE build spec" ("Selection warning")) -> (error out=w405:errorcluster)  [unwired: 1 in, 1 out]
      }
      frame "Populate Package List" {
        # "Populate Package List"
        n180 = property on="Measurement List" class="LstBox (strict)"(error in=w433) -> (error out=w420:errorcluster, "Item Names"=w432:string[], "Item Symbols"=w431:i32[])  [unwired: 1 in, 1 out]
        n181 = call "Project Path Getter.vi"("error in (no error)"=w420) -> ("Path"=w418:path, "error out"=w419:errorcluster)  [unwired: 13 in]
        n182 = for {
          tunnel: w432 -> [w437] mode=indexing
          tunnel: w431 -> [w441] mode=indexing
          tunnel: [w437] -> w430 mode=indexing if=w436
          tunnel: [w440] -> w422 mode=indexing if=w436
          shift-right: [w438] -> w429
          shift-left: w419 -> [w439]
          tunnel: w418 -> [w434]
          n183 = call "Icons.vi"() -> ("Selected"=w435:i32)  [unwired: 14 in, 1 out]
          n184 = Equal?(x=w441, y=w435) -> (x = y?=w436:bool)
          n185 = case shown="True" w436 {
            tunnel: [_ w449] -> w440
            tunnel: w439 -> [w442 w454]
            tunnel: [w442 w451] -> w438
            tunnel: w437 -> [_ w455]
            tunnel: w434 -> [_ w453]
            frame False {
            }
            frame True {
              n186 = call-poly <vilib>:"Get Build Specification Version.vi"("error in (no error)"=w454, "Name of build specification"=w455, "Path to project"=w453) -> ("error out"=w450:errorcluster, "Build Specification Version"=w444:T10)  [unwired: 7 in]
              n187 = call "Check Initial Version.vi"("Build Version In"=w444) -> ("Build Version Out"=w443:T10)  [unwired: 14 in]
              n188 = Unbundle By Name(w443) -> ("Major"=w448:u16, "Minor"=w447:u16, "Fix"=w446:u16, "Build"=w445:u16)
              n189 = Format Into String(format string="%d.%d.%d.%d", error in=w450, w448, w447, w446, w445) -> (resulting string=w449:string, error out=w451:errorcluster)  [unwired: 1 in]
            }
          }
        }
        n190 = Build Array(w430, w422) -> (w426:string[][])
        n191 = Transpose 2D Array(2D array=w426) -> (transposed array=w423:string[][])
        n192 = property on="Package List" class="MCListbox (strict)"(error in=w429, "ItemNames"=w423, "SelMode"=0 ("Selection Mode")) -> (error out=w428:errorcluster)  [unwired: 1 in, 1 out]
        n193 = Bundle By Name(cluster=w421, "Package Details"=w423) -> (w424:T7)
        n194 = property on="Tab Control" class="TabCtl (strict)"(error in=w428, "Value"=T1."Packages" ("Tab Control")) -> (error out=w427:errorcluster)  [unwired: 1 in, 1 out]
      }
      frame "Validate Configuration" {
        w458 = FALSE ("Visible")
        # "Check if configuration maintainer, maintainer email ID is valid"
        n195 = call "Queue Driver.vi"("States[]"=string[] ["Filter the Selected Measurements", "Build", "Post Build"], "error in (no error)"=w462, "Q Operations"=Queue_Operations."Enqueue N") -> ("error out"=w459:errorcluster)  [unwired: 11 in, 1 out]
        n196 = property on="Settings Page" class="TabCtl (strict)"(error in=w459, "Visible"=w458) -> (error out=w457:errorcluster)  [unwired: 1 in, 1 out]
        n197 = property on="Maintainer Warning" class="Str"(error in=w457, "Visible"=w458) -> (error out=w461:errorcluster)  [unwired: 1 in, 1 out]
      }
      frame "Filter the Selected Measurements" {
        # "Get the selected measurements"
        n198 = property on="Measurement List" class="LstBox (strict)"(error in=w472) -> (error out=w469:errorcluster, "Item Names"=w470:string[], "Item Symbols"=w471:i32[])  [unwired: 1 in, 1 out]
        n199 = Unbundle By Name(w466) -> ("Build Spec"=w467:T9[])
        n200 = call "Get Selected Meas Data.vi"("Build Spec"=w467, "Item Names"=w470, "Item Symbols"=w471, "error in (no error)"=w469) -> ("Selected Meas"=w465:T9[], "error out"=w468:errorcluster)  [unwired: 10 in]
        n201 = Bundle By Name(cluster=w466, "Selected Meas"=w465) -> (w464:T7)
      }
      frame "Post Edit Validation" {
        # "After editing validate if the changes are valid"
        n202 = Unbundle By Name(w488) -> ("Package Details"=w486:string[][])
        n203 = property on="Package List" class="MCListbox (strict)"(error in=w487) -> (error out=w480:errorcluster, "ItemNames"=w484:string[][])  [unwired: 1 in, 1 out]
        n204 = Index Array(array=w486, index (col) #1=0 ("disabled index (col)"), index (col) #2=1 ("disabled index (col)")) -> (element #1=w481:string[], element #2=w474:string[])  [unwired: 2 in]
        n205 = Index Array(array=w484, index (col)=1 ("disabled index (col)")) -> (element=w473:string[])  [unwired: 1 in]
        n206 = call "Validate the version.vi"("Old Version"=w474, "New Version"=w473, "error in (no error)"=w480) -> ("Version Out"=w475:string[], "error out"=w479:errorcluster)  [unwired: 11 in]
        n207 = Build Array(w481, w475) -> (w476:string[][])
        n208 = Transpose 2D Array(2D array=w476) -> (transposed array=w477:string[][])
        n209 = property on="Package List" class="MCListbox (strict)"(error in=w479, "ItemNames"=w477) -> (error out=w478:errorcluster)  [unwired: 1 in, 1 out]
      }
      frame "Build" {
        # "Start build process"
        n210 = property on="Tab Control" class="TabCtl (strict)"(error in=w506, "Value"=T1."Progress" ("Tab Control")) -> (error out=w502:errorcluster)  [unwired: 1 in, 1 out]
        n211 = property on="Progres Bar" class="Slide (strict)"(error in=w502, "Value"=2 ("Progres Bar")) -> (error out=w503:errorcluster)  [unwired: 1 in, 1 out]
        n212 = Unbundle By Name(w499) -> ("Build Packge?"=w493:bool, "Open Directory?"=w492:bool, "Feed"=w491:T2, "Feed Path"=w490:path, "Selected Meas"=w489:T9[])
        n213 = property on="Package List" class="MCListbox (strict)"(error in=w503) -> (error out=w498:errorcluster, "ItemNames"=w497:string[][])  [unwired: 1 in, 1 out]
        n214 = control-ref of="Progres Bar"() -> (w494:refnum<vi>)
        n215 = call "Start Build.vi"("Open Directory?"=w492, "Build Packge?"=w493, "Progres Bar"=w494, "Feed"=w491, "Feed Path"=w490, "Selected Meas"=w489, "error in (no error)"=w498, "Package Spec"=w497) -> ("Status"=w495:string[], "error out"=w496:errorcluster)  [unwired: 6 in]
        n216 = Bundle By Name(cluster=w499, "Status"=w495) -> (w505:T7)
        n217 = property on="Tab Control" class="TabCtl (strict)"(error in=w496, "Value"=T1."Next Steps" ("Tab Control")) -> (error out=w507:errorcluster)  [unwired: 1 in, 1 out]
      }
      frame "Post Build" {
        # "Populate the results in post build"
        n218 = Unbundle By Name(w514) -> ("Selected Meas"=w513:T9[], "Status"=w508:string[])
        n219 = for {
          tunnel: w513 -> [w518] mode=indexing
          tunnel: [w517] -> w512 mode=indexing
          tunnel: [""] -> _ mode=indexing
          n220 = Unbundle By Name(w518) -> ("EXE Name"=w517:string)
        }
        n221 = Build Array(w512, w508) -> (w511:string[][])
        n222 = Transpose 2D Array(2D array=w511) -> (transposed array=w510:string[][])
        n223 = property on="Build Status" class="MCListbox (strict)"(error in=w509, "ItemNames"=w510) -> (error out=w515:errorcluster)  [unwired: 1 in, 1 out]
      }
      frame "Error" {
        n224 = call <vilib>:"Simple Error Handler.vi"("error in (no error)"=w526) -> ("error out"=w519:errorcluster)  [unwired: 4 in, 4 out]
        n225 = call <vilib>:"Clear Errors.vi"("error in (no error)"=w519) -> ("error out"=w522:errorcluster)  [unwired: 5 in, 1 out]
        n226 = call "Queue Driver.vi"("error in (no error)"=w522, "Q Operations"=Queue_Operations."Flush") -> ("error out"=w521:errorcluster)  [unwired: 12 in, 1 out]
        n227 = call "Queue Driver.vi"("State"="Exit", "error in (no error)"=w521, "Q Operations"=Queue_Operations."Enqueue") -> ("error out"=w525:errorcluster)  [unwired: 11 in, 1 out]
      }
      frame "Exit" {
        n228 = call "Queue Driver.vi"("error in (no error)"=w532, "Q Operations"=Queue_Operations."Flush") -> ("error out"=w530:errorcluster)  [unwired: 12 in, 1 out]
        n229 = call "Queue Driver.vi"("error in (no error)"=w530, "Q Operations"=Queue_Operations."Release") -> ("error out"=w531:errorcluster)  [unwired: 12 in, 1 out]
      }
    }
  }
  n230 = invoke class="VI" method="FP.Close"(error in=w5) -> (error out=→"error out":errorcluster)  [unwired: 2 in, 2 out]
